vi "rad_Open Session.vi"(6 "Timeout ms (4s)":u32=4000, 7 "User name":string="admin", 8 "error in (no error)":errorcluster, 11 "Target Address":string) -> (0 "error out":errorcluster, 1 "Password Out":string, 2 "Cancelled":bool, 3 "session out":refnum<k21>)   [LabVIEW 2013]
uses:
  <vilib>/nisyscfg/Close (System).vi
  <vilib>/nisyscfg/nisyscfg.lvlib
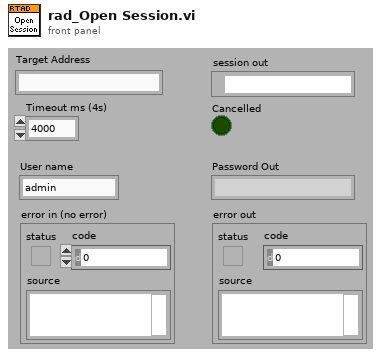
[diagram p1: front panel]
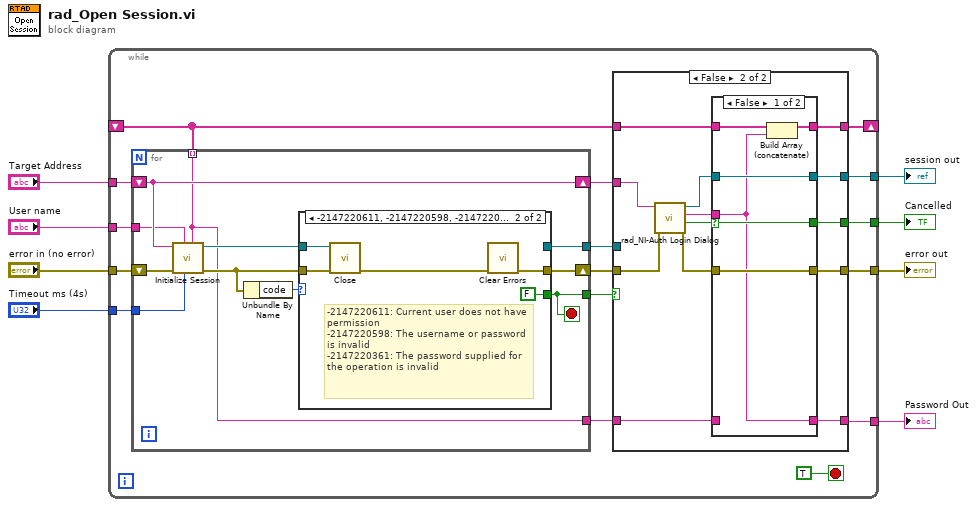
[diagram p0: block diagram]
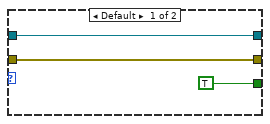
[diagram p4: hidden frame]
diagram:
  n1 = while {
    shift-right: [w15] -> _
    shift-left: _ -> [w23]
    tunnel: [w19] -> w5
    tunnel: "Target Address" -> [w18]
    tunnel: [w16] -> w7
    tunnel: [w14] -> w6
    tunnel: "error in (no error)" -> [w13]
    tunnel: "Timeout ms (4s)" -> [w12]
    tunnel: [w10] -> w2
    tunnel: "User name" -> [w9]
    stop <- TRUE stop-if-true
    n2 = for {
      tunnel: w23 -> [w53] mode=indexing
      tunnel: [w58] -> w24
      tunnel: [w57] -> w21
      shift-right: [w56] -> w17
      shift-left: w18 -> [w56]
      shift-right: [w59] -> w22
      shift-left: w13 -> [w55]
      tunnel: w12 -> [w54]
      tunnel: [w53] -> w11
      tunnel: w9 -> [w52]
      stop <- w57 stop-if-true
      n3 = call <vilib>:"Initialize Session.vi"("Password"=w53, "Connect Timeout (4000 ms)"=w54, "User Name"=w52, "error in (no error)"=w55, "Target (localhost)"=w56) -> ("error out"=w60:errorcluster, "Session out"=w62:refnum<k21>)  [unwired: 5 in]
      n4 = Unbundle By Name(w60) -> ("code"=w61:i32)
      n5 = case shown="-2147220611, -2147220598, -2147220361" w61 {
        tunnel: w62 -> [w65 w70]
        tunnel: w60 -> [w64 w69]
        tunnel: [w64 w66] -> w59
        tunnel: [w65 _] -> w58
        tunnel: [TRUE FALSE] -> w57
        frame Default {
        }
        frame -2147220611, -2147220598, -2147220361 {
          # "-2147220611: Current user does not have permission\n-2147220598: The username or password is invalid \n-2147220361: The password supplied for the operation is invalid"
          n6 = call-poly <vilib>:"Close.vi"("error in (no error)"=w69, "Session in"=w70) -> ("error out"=w67:errorcluster)  [unwired: 9 in]
          n7 = call <vilib>:"Clear Errors.vi"("error in (no error)"=w67) -> ("error out"=w66:errorcluster)  [unwired: 6 in]
        }
      }
    }
    n8 = case shown="False" w21 {
      tunnel: w24 -> [w28 _]
      tunnel: w23 -> [w27 w37]
      tunnel: w22 -> [w29 w41]
      tunnel: [w29 w32] -> w19
      tunnel: w17 -> [_ w42]
      tunnel: [FALSE w39] -> w16
      tunnel: [w27 w36] -> w15
      tunnel: [w28 w34] -> w14
      tunnel: w11 -> [w25 w30]
      tunnel: [w25 w31] -> w10
      frame True {
      }
      frame False {
        n9 = call "rad_NI-Auth Login Dialog.vi"("error in (no error)"=w41, "Target Address"=w42) -> ("error out"=w33:errorcluster, "Cancelled"=w40:bool, "Password Out"=w38:string, "session out"=w35:refnum<k21>)  [unwired: 6 in]
        n10 = case shown="False" w40 {
          selector: w40 -> [w46 w51]
          tunnel: [w46 w51] -> w39
          tunnel: w38 -> [w43 _]
          tunnel: w37 -> [w48 w50]
          tunnel: [w47 w50] -> w36
          tunnel: w35 -> [w45 _]
          tunnel: [w45 _] -> w34
          tunnel: w33 -> [w44 w49]
          tunnel: [w44 w49] -> w32
          tunnel: [w43 _] -> w31
          tunnel: w30 -> [_ _]
          frame False {
            n11 = Build Array (concatenate)(w48, w43) -> (w47:string[])
          }
          frame True {
          }
        }
      }
    }
  }
  "Cancelled" <- w7
  "session out" <- w6
  "error out" <- w5
  "Password Out" <- w2
